vi "TestExec.Get Route Config.vi"(9 "Station Name":string, 11 "Sta Config INI":path) -> (1 "Route File":path, 2 "OK":bool, 3 "Routes":string[](array[string]))   [LabVIEW 2018]
uses:
  <vilib>/Utility/config.llb/Read Key (String).vi
  <vilib>/Utility/config.llb/NI_LVConfig.lvlib
  <vilib>/KATE/Files/File Utils.lvlib
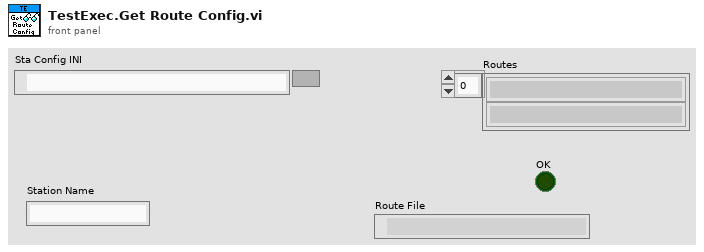
[diagram p1: front panel]
types:
  T1 = cluster{"Route File":path, "Routes":string[], "OK":bool}
  T2 = typedef "NI_LVConfig.lvlib/Config Data RefNum.ctl" = refnum<k1>
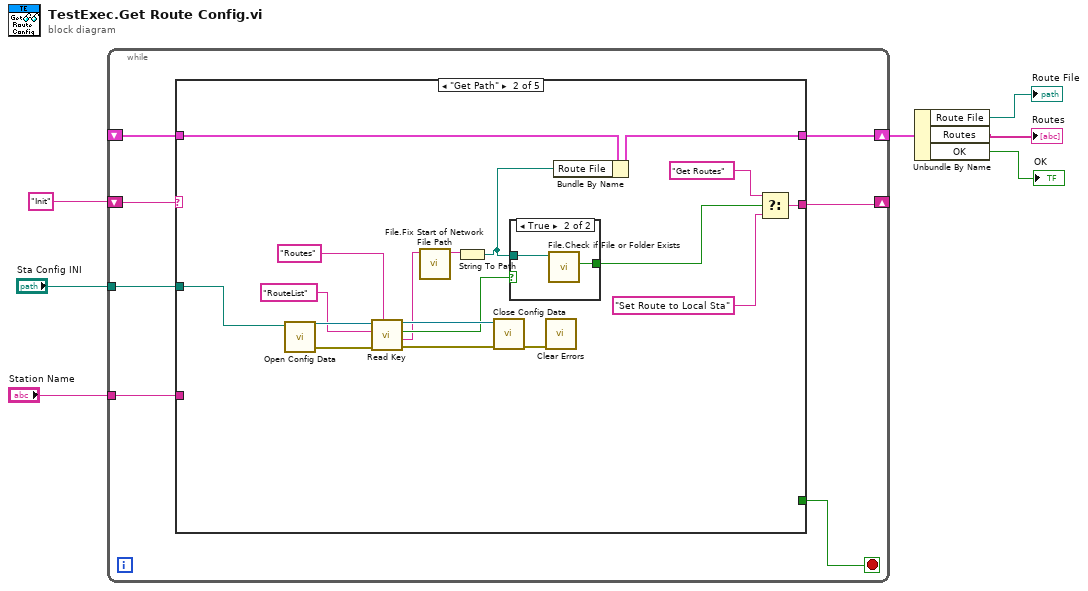
[diagram p0: block diagram]
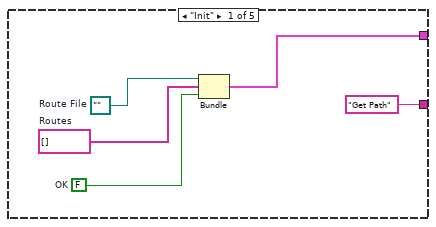
[diagram p2: hidden frame]
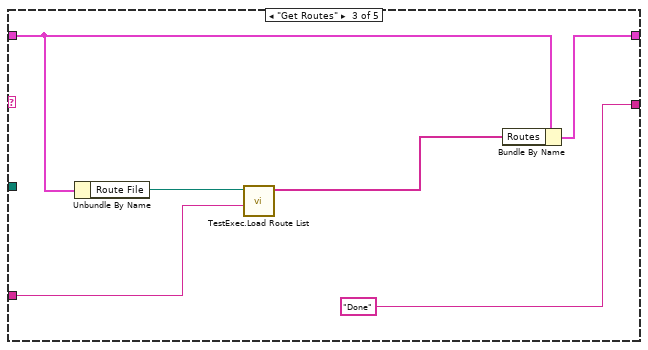
[diagram p4: hidden frame]
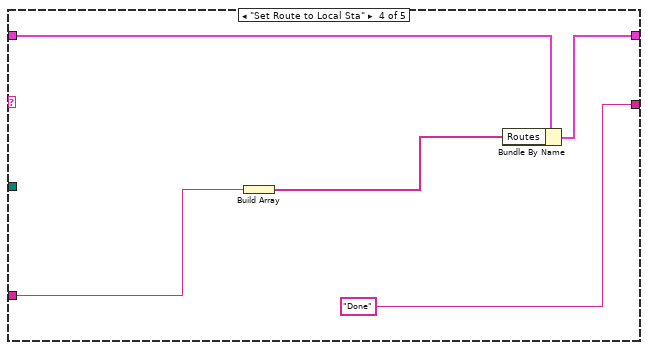
[diagram p5: hidden frame]
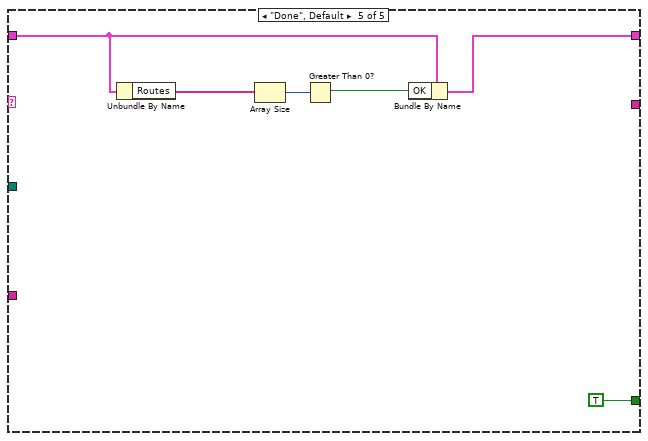
[diagram p6: hidden frame]
diagram:
  n1 = while {
    tunnel: "Sta Config INI" -> [w9]
    shift-right: [w12] -> w5
    shift-left: _ -> [w13]
    shift-right: [w11] -> _
    shift-left: "Init" -> [w14]
    tunnel: "Station Name" -> [w8]
    stop <- w10 stop-if-true
    n2 = case shown="\"Get Path\"" w14 {
      tunnel: w13 -> [_ w37 w45 w50 w54]
      tunnel: [w18 w36 w44 w49 w55] -> w12
      tunnel: ["Get Path" w25 "Done" ("format string") "Done" ("format string") _] -> w11
      tunnel: [_ _ _ _ TRUE] -> w10
      tunnel: w9 -> [_ w35 _ _ _]
      tunnel: w8 -> [_ _ w40 w46 _]
      frame "Init" {
        w16 = FALSE  # OK
        w19 = string[] []  # Routes
        w15 = path ""  # Route File
        n3 = Bundle("Route File"=w15, "Routes"=w19, "OK"=w16) -> (w18:T1)  [unwired: 1 in]
      }
      frame "Get Path" {
        n4 = call <vilib>:"Open Config Data.vi"("configuration file path"=w35) -> ("error out"=w33:errorcluster, "refnum"=w34:T2)  [unwired: 8 in, 1 out]
        n5 = call-poly <vilib>:"Read Key.vi"("section"="Routes" ("key"), "error in (no error)"=w33, "key"="RouteList", "refnum"=w34) -> ("error out"=w29:errorcluster, "value"=w22:string, "found?"=w24:bool, "refnum out"=w30:T2)  [unwired: 4 in]
        n6 = call "File.Fix Start of Network File Path.vi"("String Path"=w22) -> ("String Path Out"=w21:string)  [unwired: 10 in]
        n7 = String To Path(string=w21) -> (path=w20:path)
        n8 = call <vilib>:"Close Config Data.vi"("error in (no error)"=w29, "refnum"=w30) -> ("error out"=w28:errorcluster)  [unwired: 8 in, 1 out]
        n9 = case shown="True" w24 {
          tunnel: w20 -> [_ w39]
          tunnel: [_ w38] -> w23
          frame False {
          }
          frame True {
            n10 = call <vilib>:"File.Check if File or Folder Exists.vi"("Path"=w39) -> ("Exists"=w38:bool)  [unwired: 6 in, 4 out]
          }
        }
        n11 = call <vilib>:"Clear Errors.vi"("error in (no error)"=w28) -> ()  [unwired: 5 in, 2 out]
        n12 = Bundle By Name(cluster=w37, "Route File"=w20) -> (w36:T1)
        n13 = Select(t="Get Routes", s=w23, f="Set Route to Local Sta") -> (s? t:f=w25:string)
      }
      frame "Get Routes" {
        n14 = Unbundle By Name(w45) -> ("Route File"=w42:path)
        n15 = call "TestExec.Load Route List.vi"("Station Name"=w40, "Route List File"=w42) -> ("Route List"=w41:string[])  [unwired: 9 in]
        n16 = Bundle By Name(cluster=w45, "Routes"=w41) -> (w44:T1)
      }
      frame "Set Route to Local Sta" {
        n17 = Build Array(w46) -> (w47:string[])
        n18 = Bundle By Name(cluster=w50, "Routes"=w47) -> (w49:T1)
      }
      frame "Done", Default {
        n19 = Unbundle By Name(w54) -> ("Routes"=w53:string[])
        n20 = Array Size(array=w53) -> (size(s)=w52:i32)
        n21 = Greater Than 0?(x=w52) -> (x > 0?=w51:bool)
        n22 = Bundle By Name(cluster=w54, "OK"=w51) -> (w55:T1)
      }
    }
  }
  n23 = Unbundle By Name(w5) -> ("Route File"=→"Route File":path, "Routes"=→"Routes":string[], "OK"=→"OK":bool)
